vi "Get Reference for Specified Type (Target).vi"(8 "error in (no error)":errorcluster, 10 "Item to Find":string, 11 "Array of References":refnum<vi>[](array[refnum])) -> (0 "error out":errorcluster, 2 "Item Found":bool, 3 "TargetItem out":refnum<vi>)   [LabVIEW 2014, in "SPI Engine Scripting.lvlib"]
uses:
  SPI Engine Scripting.lvlib
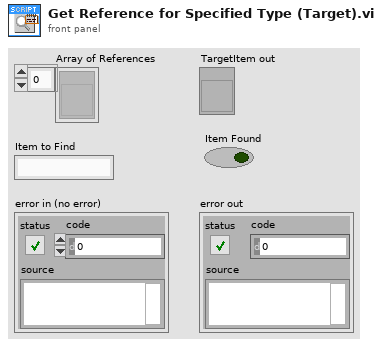
[diagram p1: front panel]
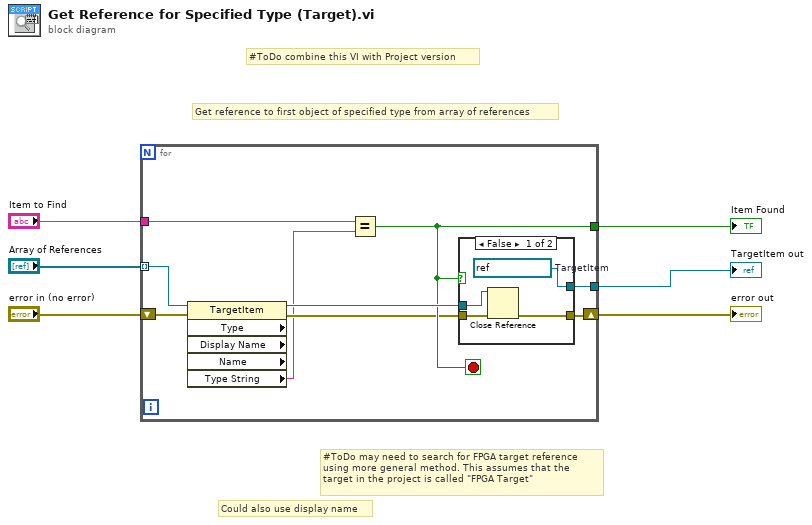
[diagram p0: block diagram]
diagram:
  # "#ToDo combine this VI with Project version"
  # "#ToDo may need to search for FPGA target reference\nusing more general method. This assumes that the\ntarget in the project is called \"FPGA Target\""
  # "Could also use display name"
  # "Get reference to first object of specified type from array of references"
  n1 = for {
    tunnel: "Array of References" -> [w15] mode=indexing
    tunnel: "Item to Find" -> [w12]
    tunnel: [w11] -> w5
    shift-right: [w9] -> w1
    shift-left: "error in (no error)" -> [w14]
    tunnel: [w8] -> w6
    stop <- w11 stop-if-true
    n2 = property class="TargetItem" props=["Type", "Display Name", "Name", "Type String"](reference=w15, error in=w14) -> (reference out=w13:refnum<vi>, error out=w10:errorcluster, "Type String"=w7:string)  [unwired: 3 out]
    n3 = Equal?(x=w12, y=w7) -> (x = y?=w11:bool)
    n4 = case shown="False" w11 {
      tunnel: w13 -> [w17 w21]
      tunnel: [w16 w21] -> w8
      tunnel: w10 -> [w19 w20]
      tunnel: [w18 w20] -> w9
      frame False {
        w16 = refnum<vi> refnum  # TargetItem
        n5 = Close Reference(reference=w17, error in (no error)=w19) -> (error out=w18:errorcluster)
      }
      frame True {
      }
    }
  }
  "TargetItem out" <- w6
  "error out" <- w1
  "Item Found" <- w5
